vi "Switch Configuration - Update Channel List in VeriStand.vi"(8 "error in (no error)":errorcluster, 10 "Item Names":string[](array[string]), 11 "Item Ref In":T1 format="%.0x") -> (0 "error out":errorcluster, 3 "Item Ref Out":T1=18446744073709551615 format="%.0x")   [LabVIEW 2015, in "DMM-SWITCH-ScanList System Explorer.lvlib"]
doc: "Update Measurement Channels in VeriStand. Deletes current Measurement Channels and creates new Measurement Channels based on updated Switch Configuration"
uses:
  DMM-SWITCH-ScanList System Explorer.lvlib
  <vilib>/NI Veristand/Custom Device API/Custom Device Item Ref.ctl
  <vilib>/NI Veristand/Custom Device API/Custom Device Channel Type.ctl
  <vilib>/NI Veristand/Custom Device API/Custom Device Channel.ctl
  Shared/Constants.vi
  <vilib>/NI Veristand/Custom Device API/Custom Device API.lvlib
  Shared/DMM-SWITCH-ScanList Shared.lvlib
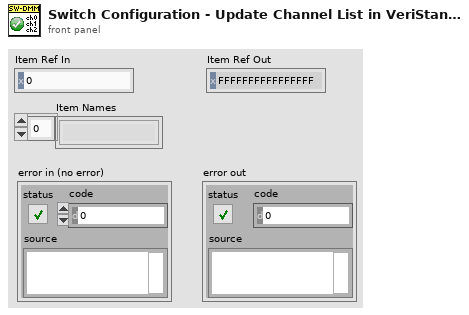
[diagram p1: front panel]
types:
  T1 = typedef "Custom Device API.lvlib/Custom Device Item Ref.ctl" = u64
  T2 = typedef "Custom Device API.lvlib/Custom Device Channel.ctl" = cluster{"Type":T3, "Units":string, "Default Value":dbl, "Faultable":bool, "Scalable":bool}
  T3 = typedef "Custom Device API.lvlib/Custom Device Channel Type.ctl" = enum16{"Input", "Output"}
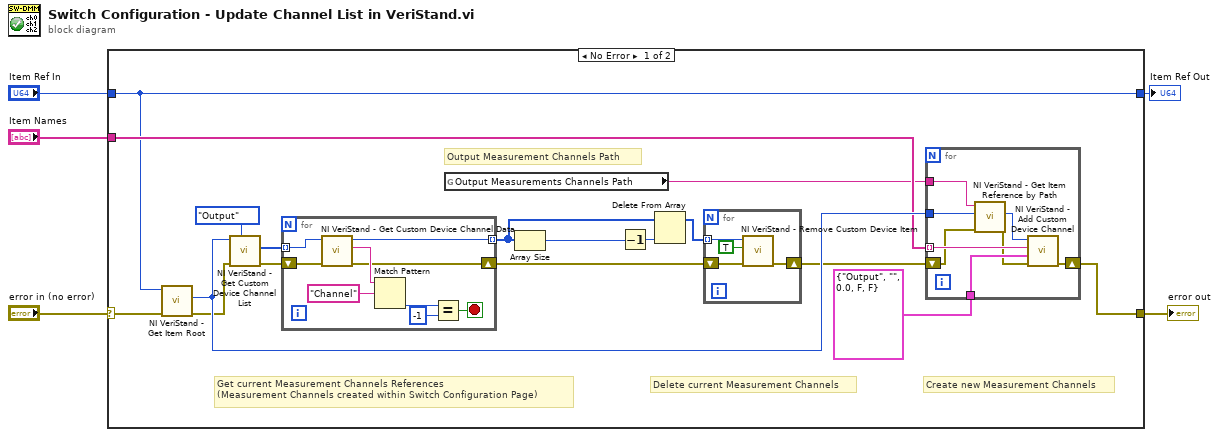
[diagram p0: block diagram]
diagram:
  n1 = case shown="No Error" "error in (no error)" {
    selector: "error in (no error)" -> [w9 w45]
    tunnel: [w18 w45] -> w5
    tunnel: "Item Ref In" -> [w7 w44]
    tunnel: "Item Names" -> [w8 _]
    tunnel: [w7 w44] -> w1
    frame No Error {
      # "Output Measurement Channels Path"
      # "Create new Measurement Channels"
      # "Delete current Measurement Channels"
      # "Get current Measurement Channels References\n(Measurement Channels created within Switch Configuration Page)"
      n2 = call <vilib>:"NI VeriStand - Get Item Root.vi"("error in (no error)"=w9, "Item Ref in"=w7) -> ("error out"=w12:errorcluster, "Root Ref out"=w21:T1)  [unwired: 6 in, 2 out]
      n3 = call <vilib>:"NI VeriStand - Get Custom Device Channel List.vi"("Channel Type"=Custom_Device_Channel_Type."Output", "error in (no error)"=w12, "Device Ref in"=w21) -> ("error out"=w13:errorcluster, "Specified Channel Ref List"=w11:T1[])  [unwired: 6 in, 1 out]
      n4 = for {
        tunnel: w11 -> [w43] mode=indexing
        shift-right: [w36] -> w22
        shift-left: w13 -> [w41]
        tunnel: [w35] -> w14 mode=indexing
        stop <- w38 stop-if-true
        n5 = call <vilib>:"NI VeriStand - Get Custom Device Channel Data.vi"("error in (no error)"=w41, "Channel Ref in"=w43) -> ("error out"=w36:errorcluster, "Channel Name"=w37:string, "Channel Ref out"=w35:T1)  [unwired: 4 in, 3 out]
        n6 = Match Pattern(string=w37, regular expression="Channel") -> (offset past match=w40:i32)  [unwired: 1 in, 3 out]
        n7 = Equal?(x=w40, y=-1) -> (x = y?=w38:bool)
      }
      n8 = global read "Constants.vi" "Output Measurements Channels Path"() -> (w6:string)
      n9 = Array Size(array=w14) -> (size(s)=w15:i32)
      n10 = Decrement(x=w15) -> (x-1=w16:i32)
      n11 = Delete From Array(array=w14, index=w16) -> (array with subset deleted=w19:T1[])  [unwired: 1 in, 1 out]
      n12 = for {
        tunnel: w19 -> [w34] mode=indexing
        shift-right: [w31] -> w20
        shift-left: w22 -> [w32]
        n13 = call <vilib>:"NI VeriStand - Remove Custom Device Item.vi"("error in (no error)"=w32, "Force Delete (F)"=TRUE, "Item Ref in"=w34) -> ("error out"=w31:errorcluster)  [unwired: 7 in, 1 out]
      }
      n14 = for {
        tunnel: T2 {"Type"=enum."Output", "Units"="", "Default Value"=0.0, "Faultable"=FALSE, "Scalable"=FALSE} ("Channel") -> [w30]
        tunnel: w8 -> [w27] mode=indexing
        shift-right: [w29] -> w18
        shift-left: w20 -> [w26]
        tunnel: w21 -> [w24]
        tunnel: w6 -> [w23]
        n15 = call <vilib>:"NI VeriStand - Get Item Reference by Path.vi"("error in (no error)"=w26, "Root Ref"=w24, "Item Path in"=w23) -> ("error out"=w25:errorcluster, "Item Ref"=w28:T1)  [unwired: 5 in, 2 out]
        n16 = call <vilib>:"NI VeriStand - Add Custom Device Channel.vi"("error in (no error)"=w25, "Channel"=w30, "Channel Name"=w27, "Parent Ref in"=w28) -> ("error out"=w29:errorcluster)  [unwired: 4 in, 3 out]
      }
    }
    frame Error {
    }
  }
  "error out" <- w5
  "Item Ref Out" <- w1
